vi "ConvertVariousStrToByteArr.vi"(10 "various type":enum16{"hex", "asc"}(ring), 11 "various str":string) -> (3 "data out":u8[](array[numeric]))   [LabVIEW 2018, in "Library-DataConvert.lvlib"]
uses:
  Library-DataConvert.lvlib
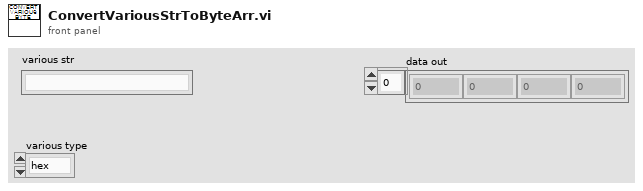
[diagram p1: front panel]
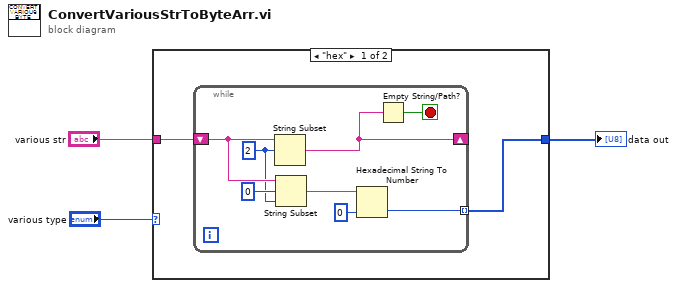
[diagram p0: block diagram]
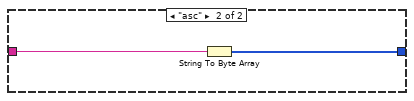
[diagram p2: hidden frame]
diagram:
  n1 = case shown="\"hex\"" "various type" {
    tunnel: "various str" -> [w5 w15]
    tunnel: [w4 w14] -> w1
    frame "hex" {
      n2 = while {
        shift-right: [w12] -> _
        shift-left: w5 -> [w13]
        tunnel: [w6] -> w4 mode=indexing
        stop <- w11 stop-if-true
        w9 = 2 ("오프셋(0)")
        n3 = String Subset(string=w13, offset (0)=w9) -> (substring=w12:string)  [unwired: 1 in]
        n4 = String Subset(string=w13, offset (0)=0 ("오프셋(0)"), length (rest)=w9) -> (substring=w8:string)
        n5 = Hexadecimal String To Number(string=w8, default (0uL)=u8 0 ("기본(0 U32)")) -> (number=w6:u8)  [unwired: 1 in, 1 out]
        n6 = Empty String/Path?(string/path=w12) -> (empty?=w11:bool)
      }
    }
    frame "asc" {
      n7 = String To Byte Array(string=w15) -> (unsigned byte array=w14:u8[])
    }
  }
  "data out" <- w1
